vi "VISP Draw Snippet Image.vi"(8 "error in (no error)":errorcluster, 11 "VI Refnum in":refnum<vi>) -> (0 "error out":errorcluster, 2 "Image Data":T1, 3 "dup VI Refnum":refnum<vi>)   [LabVIEW 2019, in "VI Snippet.lvlib"]
doc: "Draws the VI Snippet image from the <b>VI Refnum in</b> diagram content.\n\nCreated by: Ryan Pacini"
uses:
  VI Snippet.lvlib
  <vilib>/picture/picture.llb/imagedata.ctl
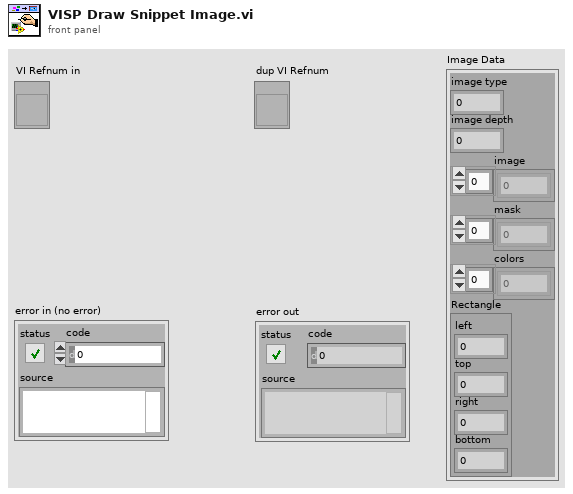
[diagram p1: front panel]
types:
  T1 = typedef "imagedata.ctl" = cluster{"image type":i32, "image depth":i32, "image":u8[], "mask":u8[], "colors":u32[], "Rectangle":cluster{"left":i16, "top":i16, "right":i16, "bottom":i16}}
  T2 = cluster{"Width":u16, "Style":enum32{"Solid", "Dash", "Dot", "DashDot", "DashDotDot"}}
  T3 = cluster{"left":i16, "top":i16, "right":i16, "bottom":i16}
  T4 = cluster{"left":i16, "top":i16, "right":i16, "bottom":i16}[]
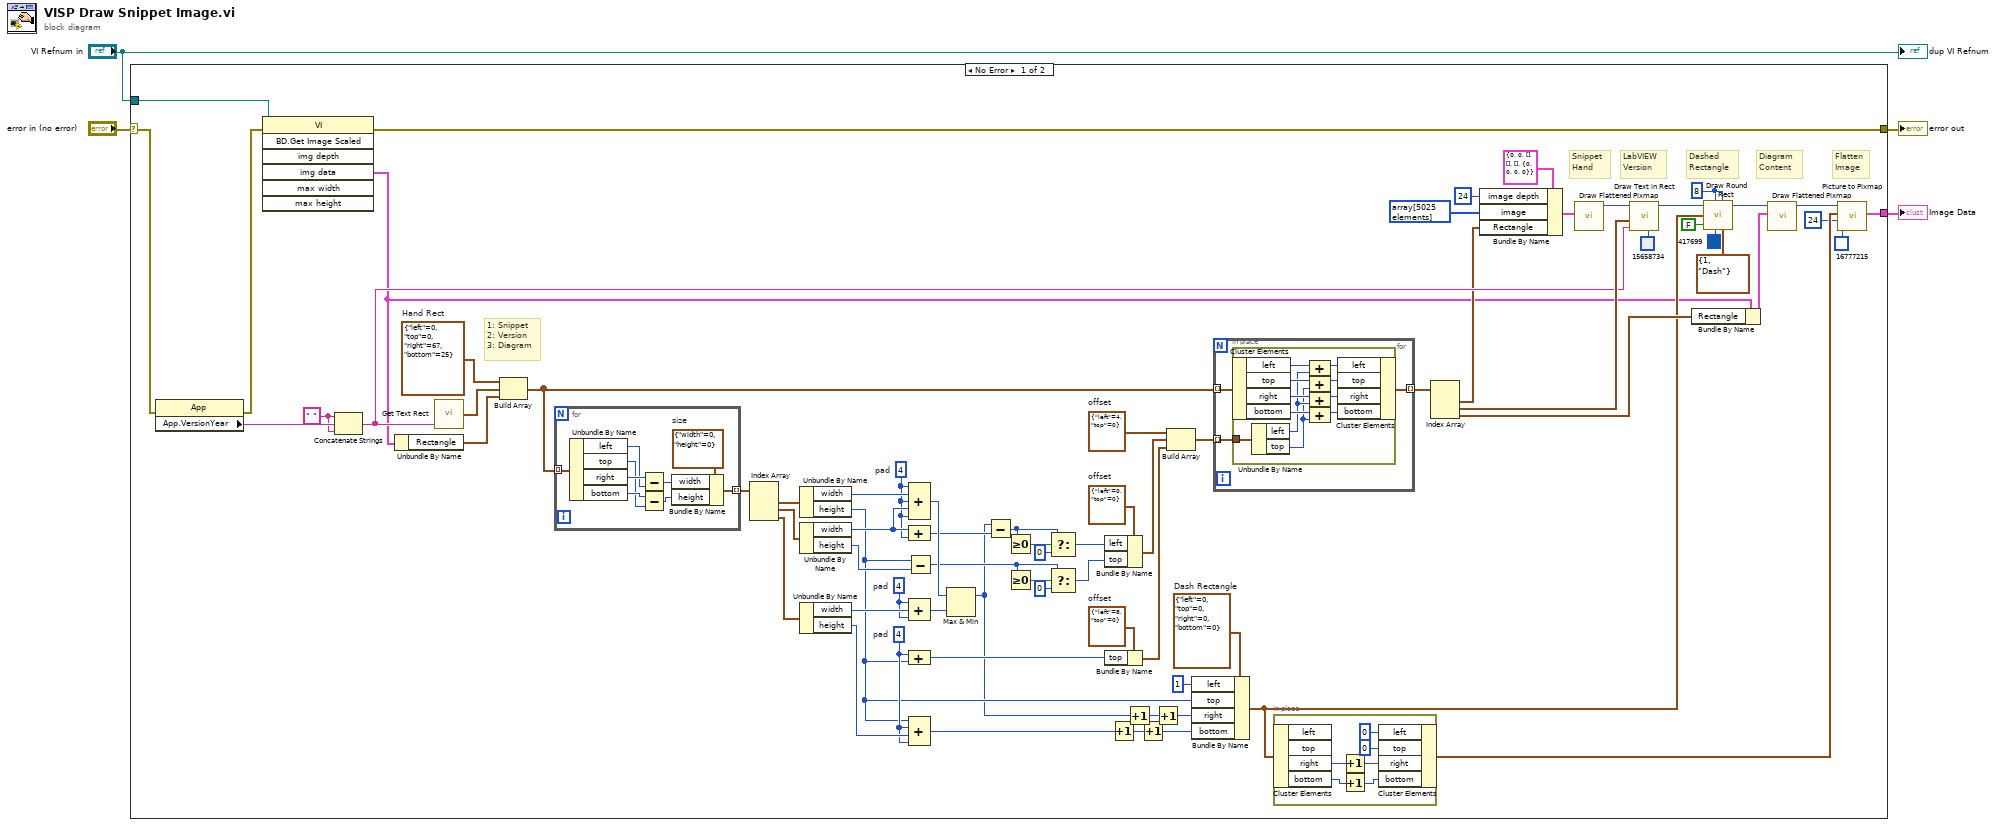
[diagram p0: block diagram]
diagram:
  n1 = case shown="No Error" "error in (no error)" {
    selector: "error in (no error)" -> [w6 w108]
    tunnel: [w7 w108] -> w3
    tunnel: "VI Refnum in" -> [w14 _]
    tunnel: [w22 _] -> w2
    frame No Error {
      w17 = T3 {"left"=0, "top"=0, "right"=67, "bottom"=25}  # Hand Rect
      w29 = " " ("string")
      w28 = i16 4  # pad
      w48 = i16 8 ("oval width")
      w40 = T3 {"left"=0, "top"=0, "right"=0, "bottom"=0}  # Dash Rectangle
      w34 = i16 4  # pad
      w39 = i16 4  # pad
      w70 = cluster{"left":i16, "top":i16} {"left"=0, "top"=0}  # offset
      w72 = cluster{"left":i16, "top":i16} {"left"=8, "top"=0}  # offset
      w73 = cluster{"left":i16, "top":i16} {"left"=4, "top"=0}  # offset
      # "Flatten\nImage"
      # "Diagram\nContent"
      # "Dashed\nRectangle"
      # "LabVIEW\nVersion"
      # "Snippet\nHand"
      # "1: Snippet\n2: Version\n3: Diagram"
      n2 = property class="App"(error in=w6) -> (error out=w5:errorcluster, "App.VersionYear"=w78:string)  [unwired: 1 in, 1 out]
      n3 = invoke class="VI" method="BD.Get Image Scaled"(reference=w14, error in=w5) -> (error out=w7:errorcluster, "img data"=w13:T1)  [unwired: 5 in, 5 out]
      n4 = Concatenate Strings(w29, w78, w29) -> (w30:string)
      n5 = Unbundle By Name(w13) -> ("Rectangle"=w74:T3)
      n6 = call <vilib>:"Get Text Rect.vi"("text"=w30) -> ("rect"=w75:T3)  [unwired: 8 in]
      n7 = Build Array(w17, w75, w74) -> (w57:T4)
      n8 = for {
        tunnel: w57 -> [w80] mode=indexing
        tunnel: [w79] -> w68 mode=indexing
        w83 = cluster{"width":i16, "height":i16} {"width"=0, "height"=0}  # size
        n9 = Unbundle By Name(w80) -> ("left"=w84:i16, "top"=w85:i16, "right"=w87:i16, "bottom"=w86:i16)
        n10 = Subtract(x=w87, y=w84) -> (x-y=w82:i16)
        n11 = Subtract(x=w86, y=w85) -> (x-y=w81:i16)
        n12 = Bundle By Name(cluster=w83, "width"=w82, "height"=w81) -> (w79:cluster{"width":i16, "height":i16})
      }
      n13 = Index Array(array=w68) -> (element #1=w67:cluster{"width":i16, "height":i16}, element #2=w66:cluster{"width":i16, "height":i16}, element #3=w64:cluster{"width":i16, "height":i16})  [unwired: 3 in]
      n14 = Unbundle By Name(w67) -> ("width"=w65:i16, "height"=w27:i16)
      n15 = Unbundle By Name(w66) -> ("width"=w60:i16, "height"=w45:i16)
      n16 = Unbundle By Name(w64) -> ("width"=w63:i16, "height"=w33:i16)
      n17 = Subtract(x=w27, y=w45) -> (x-y=w43:i16)
      n18 = Compound Arithmetic op=ADD(w39, w65, w39, w60, w39) -> (w62:i16)
      n19 = Compound Arithmetic op=ADD(w60, w39) -> (w59:i16)
      n20 = Compound Arithmetic op=ADD(w34, w63, w34) -> (w61:i16)
      n21 = Compound Arithmetic op=ADD(w28, w27) -> (w31:i16)
      n22 = Compound Arithmetic op=ADD(w27, w28, w33, w28) -> (w32:i16)
      n23 = Max & Min(x=w62, y=w61) -> (max(x,y)=w12:i16)  [unwired: 1 out]
      n24 = Subtract(x=w12, y=w59) -> (x-y=w36:i16)
      n25 = Greater Or Equal To 0?(x=w36) -> (x >= 0?=w37:bool)
      n26 = Greater Or Equal To 0?(x=w43) -> (x >= 0?=w44:bool)
      n27 = Select(t=w36, s=w37, f=i16 0) -> (s? t:f=w35:i16)
      n28 = Select(t=w43, s=w44, f=i16 0) -> (s? t:f=w41:i16)
      n29 = Bundle By Name(cluster=w70, "left"=w35, "top"=w41) -> (w69:cluster{"left":i16, "top":i16})
      n30 = Bundle By Name(cluster=w72, "top"=w31) -> (w71:cluster{"left":i16, "top":i16})
      n31 = Increment(x=w32) -> (x+1=w9:i16)
      n32 = Increment(x=w12) -> (x+1=w11:i16)
      n33 = Increment(x=w9) -> (x+1=w8:i16)
      n34 = Increment(x=w11) -> (x+1=w10:i16)
      n35 = Build Array(w73, w69, w71) -> (w58:cluster{"left":i16, "top":i16}[])
      n36 = Bundle By Name(cluster=w40, "left"=i16 1, "top"=w27, "right"=w10, "bottom"=w8) -> (w26:T3)
      n37 = for {
        tunnel: [w96] -> w76 mode=indexing
        tunnel: w58 -> [w95] mode=indexing
        tunnel: w57 -> [w94] mode=indexing
        n38 = in-place {
          in-place-border: w95 -> [w103]
          n39 = in-place-cluster #1(w94) -> ("left"=w104:i16, "top"=w105:i16, "right"=w106:i16, "bottom"=w107:i16)
          n40 = Unbundle By Name(w103) -> ("left"=w102:i16, "top"=w101:i16)
          n41 = Compound Arithmetic op=ADD(w104, w102) -> (w100:i16)
          n42 = Compound Arithmetic op=ADD(w105, w101) -> (w99:i16)
          n43 = Compound Arithmetic op=ADD(w106, w102) -> (w98:i16)
          n44 = Compound Arithmetic op=ADD(w107, w101) -> (w97:i16)
          n45 = in-place-cluster #1("left"=w100, "top"=w99, "right"=w98, "bottom"=w97) -> (w96:T3)
        }
      }
      n46 = in-place {
        n47 = in-place-cluster #2(w26) -> ("right"=w91:i16, "bottom"=w90:i16)  [unwired: 2 out]
        n48 = Increment(x=w91) -> (x+1=w88:i16)
        n49 = Increment(x=w90) -> (x+1=w89:i16)
        n50 = in-place-cluster #2("left"=i16 0, "top"=i16 0, "right"=w88, "bottom"=w89) -> (w25:T3)
      }
      n51 = Index Array(array=w76) -> (element #1=w15:T3, element #2=w55:T3, element #3=w52:T3)  [unwired: 3 in]
      n52 = Bundle By Name(cluster=T1 {"image type"=0, "image depth"=0, "image"=[], "mask"=[], "colors"=[], "Rectangle"={"left"=0, "top"=0, "right"=0, "bottom"=0}}, "image depth"=24, "image"=u8[] array[5025 elements], "Rectangle"=w15) -> (w16:T1)
      n53 = call <vilib>:"Draw Flattened Pixmap.vi"("image data"=w16) -> ("new picture"=w56:picture)  [unwired: 8 in]
      n54 = call <vilib>:"Draw Text in Rect.vi"("BG color(transparent)"=u32 15658734, "text"=w30, "rect"=w55, "picture"=w56) -> ("new picture"=w53:picture)  [unwired: 7 in]
      n55 = Bundle By Name(cluster=w13, "Rectangle"=w52) -> (w46:T1)
      n56 = call <vilib>:"Draw Round Rect.vi"("picture"=w53, "oval width"=w48, "rect"=w26, "fill?(F)"=FALSE, "color(black)"=u32 417699, "oval height"=w48, "pen"=T2 {"Width"=1, "Style"=enum."Dash"}) -> ("new picture"=w47:picture)  [unwired: 2 in]
      n57 = call <vilib>:"Draw Flattened Pixmap.vi"("image data"=w46, "picture"=w47) -> ("new picture"=w21:picture)  [unwired: 7 in]
      n58 = call <vilib>:"Picture to Pixmap.vi"("Background Color"=u32 16777215, "depth"=24, "rect"=w25, "picture"=w21) -> ("image data"=w22:T1)  [unwired: 6 in, 1 out]
    }
    frame Error {
    }
  }
  "error out" <- w3
  "Image Data" <- w2
  "dup VI Refnum" <- "VI Refnum in"
